vi "Discover Nodes.vi"(8 "error in":errorcluster, 11 "CANopen Master in":refnum<class "CANopen Master.lvclass">) -> (0 "error out":errorcluster, 3 "CANopen Master out":refnum<class "CANopen Master.lvclass">)   [LabVIEW 2024, in "CANopen Master.lvlib" / "CANopen Master.lvclass"]
uses:
  CANopen Master.lvclass
  CANopen Master.lvclass/CANopen Master.ctl
  Network Mangement/Network Mangement.lvclass
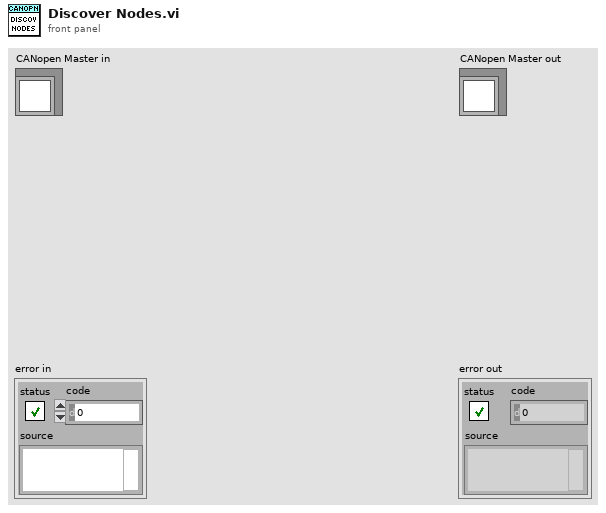
[diagram p1: front panel]
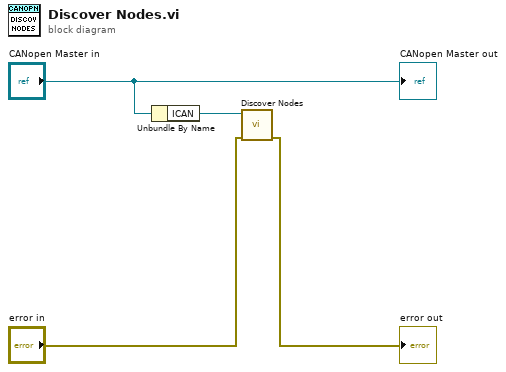
[diagram p0: block diagram]
diagram:
  n1 = Unbundle By Name("CANopen Master in") -> ("ICAN"=w3:refnum<class "ICAN.lvclass">)
  n2 = call "Discover Nodes.vi"("Error In"="error in", "ICAN"=w3) -> ("Error Out"=→"error out":errorcluster)  [unwired: 9 in]
  "CANopen Master out" <- "CANopen Master in"
